vi "WireWriteBlockDiagram.vi"(8 "error in":errorcluster, 10 "Terminal References":T4, 11 "State":T1) -> (0 "error out":errorcluster, 3 "State out":T1)   [LabVIEW 2013, in "data interface script.lvlib"]
uses:
  data interface script.lvlib
  Controls/TerminalReferences.ctl
  Controls/StateCluster.ctl
  Controls/initialized references.ctl
  Controls/interface VI type.ctl
  <vilib>/NI/Tag Bus/tag/Data Type.ctl
  <vilib>/NI/Tag Bus/tag/tag descriptor.lvclass
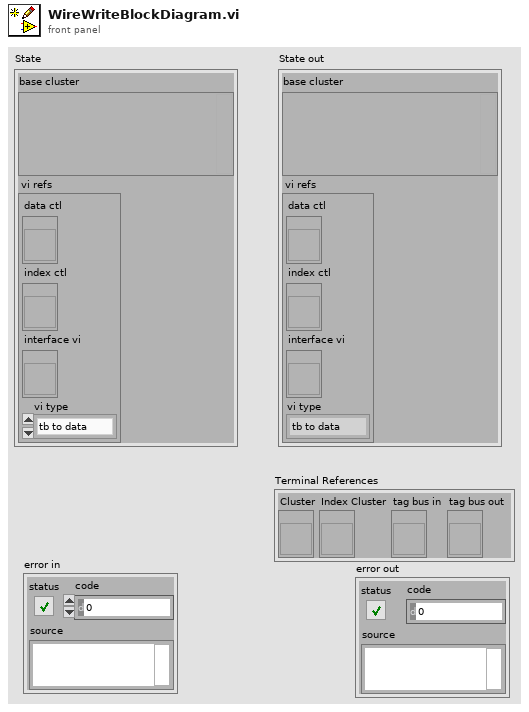
[diagram p1: front panel]
types:
  T1 = typedef "data interface script.lvlib/StateCluster.ctl" = cluster{"base cluster":variant, "vi refs":T2}
  T2 = typedef "data interface script.lvlib/initialized references.ctl" = cluster{"data ctl":refnum<vi>, "index ctl":refnum<vi>, "interface vi":refnum<vi>, "vi type":T3}
  T3 = typedef "data interface script.lvlib/interface VI type.ctl" = enum16{"tb to data", "data to tb"}
  T4 = typedef "data interface script.lvlib/TerminalReferences.ctl" = cluster{"Cluster":refnum<vi>, "Index Cluster":refnum<vi>, "tag bus in":refnum<vi>, "tag bus out":refnum<vi>}
  T5 = typedef "tag bus.lvlib/tag descriptor.lvclass/Data Type.ctl" = enum16{"Double", "Single", "I64", "I32", "I16", "I8", "U64", "U32", "U16", "U8", "Boolean", "String", "Array of Double", "Array of Single", "Array of I64", "Array of I32", "Array of I16", "Array of I8", "Array of U64", "Array of U32", "Array of U16", "Array of U8", "Array of Boolean", "Array of String"}
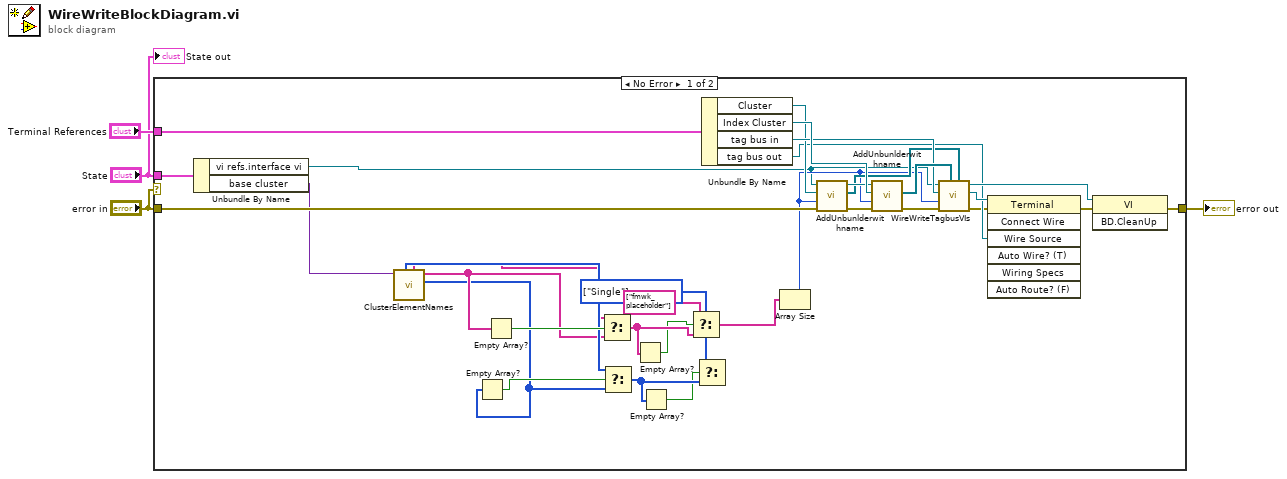
[diagram p0: block diagram]
diagram:
  n1 = case shown="No Error" "error in" {
    tunnel: "Terminal References" -> [w37 _]
    tunnel: [w36 w38] -> w3
    tunnel: "State" -> [w33 _]
    tunnel: "error in" -> [w31 w38]
    frame No Error {
      w7 = T5[] [enum."Single"] items=["Double", "Single", "I64", "I32", "I16", "I8", "U64", "U32", "U16", "U8", "Boolean", "String", "Array of Double", "Array of Single", "Array of I64", "Array of I32", "Array of I16", "Array of I8", "Array of U64", "Array of U32", "Array of U16", "Array of U8", "Array of Boolean", "Array of String"] ("t")
      n2 = Unbundle By Name(w33) -> ("vi refs.interface vi"=w20:refnum<vi>, "base cluster"=w5:variant)
      n3 = call "ClusterElementNames.vi"("input cluster"=w5) -> ("DataTypes"=w13:T5[], "Elements Names"=w14:string[], "placeholder names"=w15:string[], "placeholder types"=w16:T5[])  [unwired: 6 in, 1 out]
      n4 = Empty Array?(array=w13) -> (empty?=w17:bool)
      n5 = Empty Array?(array=w14) -> (empty?=w18:bool)
      n6 = Select(t=w15, s=w18, f=w14) -> (s? t:f=w12:string[])
      n7 = Select(t=w16, s=w17, f=w13) -> (s? t:f=w11:T5[])
      n8 = Empty Array?(array=w12) -> (empty?=w9:bool)
      n9 = Empty Array?(array=w11) -> (empty?=w10:bool)
      n10 = Select(t=string[] ["fmwk_placeholder"], s=w9, f=w12) -> (s? t:f=w6:string[])
      n11 = Select(t=w7, s=w10, f=w11) -> ()  [unwired: 1 out]
      n12 = Unbundle By Name(w37) -> ("Cluster"=w30:refnum<vi>, "Index Cluster"=w35:refnum<vi>, "tag bus in"=w32:refnum<vi>, "tag bus out"=w24:refnum<vi>)
      n13 = Array Size(array=w6) -> (size(s)=w21:i32)
      n14 = call "AddUnbunlderwithname.vi"("error in"=w31, "elements in cluster"=w21, "cluster terminal"=w30, "VI in"=w20) -> ("error out"=w28:errorcluster, "terminals"=w22:refnum<vi>[], "VI out"=w29:refnum<vi>)  [unwired: 5 in]
      n15 = call "AddUnbunlderwithname.vi"("error in"=w28, "elements in cluster"=w21, "cluster terminal"=w35, "VI in"=w29) -> ("error out"=w23:errorcluster, "terminals"=w34:refnum<vi>[])  [unwired: 5 in, 1 out]
      n16 = call "WireWriteTagbusVIs.vi"("terminals data"=w22, "terminals indexes"=w34, "error in"=w23, "elements in cluster"=w21, "tag bus in in"=w32, "VI in"=w20) -> ("error out"=w19:errorcluster, "tag bus out"=w25:refnum<vi>, "VI out"=w27:refnum<vi>)  [unwired: 3 in]
      n17 = invoke on="Invoke Node" class="Terminal" method="Connect Wire"(reference=w25, error in=w19, "Wire Source"=w24) -> (error out=w26:errorcluster)  [unwired: 4 in, 6 out]
      n18 = invoke class="VI" method="BD.CleanUp"(reference=w27, error in=w26) -> (error out=w36:errorcluster)  [unwired: 1 in, 2 out]
    }
    frame Error {
    }
  }
  "error out" <- w3
  "State out" <- "State"
